vi "PSLDAQ_GetDeviceID.vi"(1 "Handle In":T1) -> (0 "DeviceID":string)   [LabVIEW 2010]
doc: "1. 설명\n a. 통신 연결된 PSL-DAQ 장치의 장치 ID를 얻음 \n b. 참고로, 각 장치마다 고유의 장치 ID를 가짐 \n\n2. 기능\n a. PSL-DAQ 장치의 장치 ID를 얻어 문자열로 출력 \n \n3. 터미널\n a. 터미널 입력\n ○ Handle In : 장치 핸들 \n \n b. 터미널 출력\n ○ Device ID : 통신 연결된 장치의 ID \n\n4. 주의\n a. PSL-DAQ 장치와 통신 연결된 경우에 정상적으로 동작함."
uses:
  PSLDAQ_Dll.dll
panel:
  # "PSLDAQ_GetDeviceID\n\n1. 설명\n  a. 통신 연결된 PSL-DAQ 장치의 장치 ID를 얻음 \n  b. 참고로, 각 장치마다 고유의 장치 ID를 가짐 \n\n2. 기능\n  a. PSL-DAQ 장치의 장치 ID를 얻어 문자열로 출력  \n      \n3. 터미널\n  a. 터미널 입력\n     ○ Handle In : 장치 핸들 \n     \n  b. 터미널 출력\n     ○ Device ID : 통신 연결된 장치의 ID \n\n4. 주의\n  a. PSL-DAQ 장치와 통신 연결된 경우에 정상적으로 동작함."
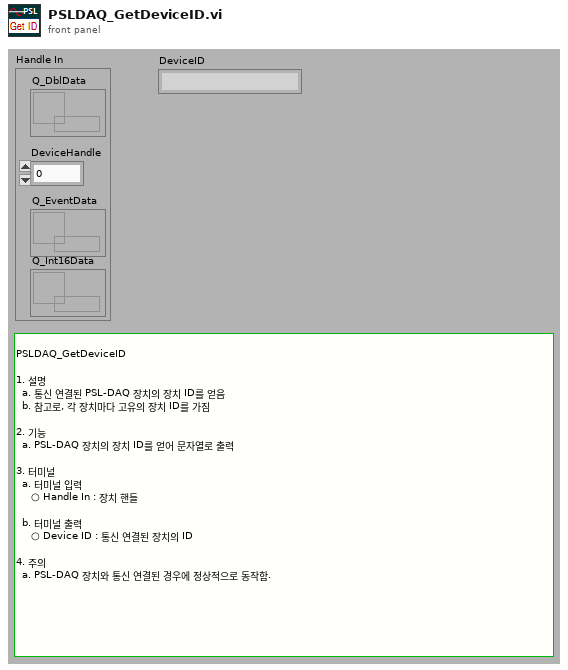
[diagram p1: front panel]
types:
  T1 = cluster{"Q_DblData":refnum<queue>, "DeviceHandle":u32, "Q_EventData":refnum<queue>, "Q_Int16Data":refnum<queue>}
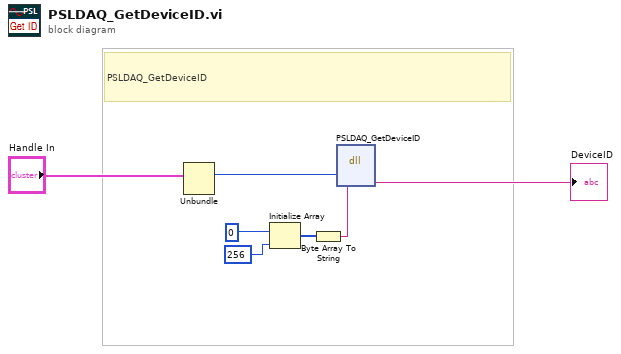
[diagram p0: block diagram]
diagram:
  # "PSLDAQ_GetDeviceID"
  n1 = Unbundle("Handle In") -> ("DeviceHandle"=w6:u32)  [unwired: 3 out]
  n2 = Initialize Array(i8 0, 256) -> (w3:i8[])
  n3 = Byte Array To String(unsigned byte array=w3) -> (string=w2:string)
  n4 = dll-call lib="D:/PSL-DAQ LabVIEW Library/PSLDAQ_Dll.dll" fn="PSLDAQ_GetDeviceID"("DeviceHandle"=w6, "DeviceID"=w2) -> ("DeviceID"=→"DeviceID":string)  [unwired: 5 in, 2 out]
